vi "CC Focus GUI.vi"(9 "Standalone":bool=TRUE, 10 "Init Data":variant, 11 "Name":string) -> ()   [LabVIEW 2024]
uses:
  typedefs/CC enum Operation Mode.ctl
  Focus cluster Settings.ctl
  Focus Hardware Types.ctl
  Focus cluster Motion Settings.ctl
  Focus Class/Focus Class.lvclass
  Subsystems/SS typedef cluster Instrument Command Queue Data.ctl
  Subsystems/SS cluster Data Queue type.ctl
  Focus cluster MoveFocus Command Parameters.ctl
  FocusSimulator/FocusSimulator.lvclass
  C:/Development/Prime-RIMAS/Focus/Focus Class/Focus Class.lvclass
  NewFocus/NewFocus.lvclass
  Focus Class/Focus Class.lvclass/Focus Class.ctl
  hk-channel-class/hk-channel-class/HK Item/HK Channel cluster Telemetry Data.ctl
  hk-channel-class/hk-channel-class/HK Item/HK Channel enum Data Type.ctl
  hk-channel-class/hk-channel-class/HK Item/HK Item.lvclass
panel:
  out "Messages":string
  in  "Mode":T1
  in  "Tab Control":T2(tab)
  in  "Absolute":bool
  in  "Relative":bool
  in  "Steps":i32
  out "Controller Name":string
  in  "Select Motor (0:n-1)":i32 min=0 max=3 step=1
  out "Positions":i32[](array[slide]) scale=-10000.0..10000.0
  in  "Error":bool
  out "Homed":bool[](array[boolean])
  in  "STOP":bool
  out "Connected":bool
  in  "Close":bool
  in  "Home":bool
  in  "Reset Startup Positions":bool
  in  "Connect":bool
  in  "Focus Settings":T3
  in  "Power Up Positions":i32[](array[numeric])
  # "The focus motors adjust the position of the detectors. These motors should only be used at room temperatures. Adjustments to focus position is for maintenance personel only. There is nothing observers need to access."
  # "Click for info"
  # "We need to remember where we were last in case\npower cycled on NewFocus controller. Change\ncode to use saved positions only if controller reports\nall 0s for position."
  # "Factory Settings: \nVelocity 1750 Steps/sec\nAcceleration 100000 Steps/sec/sec"
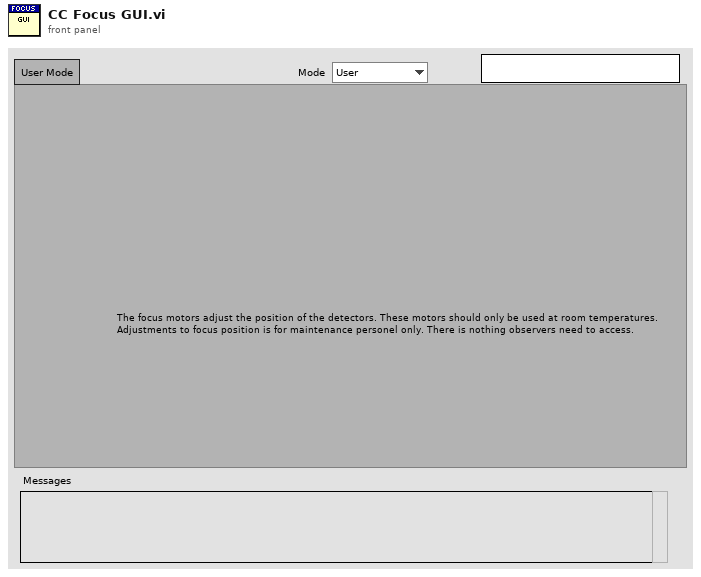
[diagram p1: front panel]
types:
  T1 = typedef "CC enum Operation Mode.ctl" = enum16{"User", "Engineering"}
  T2 = enum32{"User Mode", "Focus Motor", "Engineering"}
  T3 = typedef "Focus cluster Settings.ctl" = cluster{"Type":T4, "Motion Settings":T5, "Last Positions":i32[]}
  T4 = typedef "Focus Hardware Types.ctl" = enum16{"Simulated", "NewFocus"}
  T5 = typedef "Focus cluster Motion Settings.ctl" = cluster{"Steps Per Sec":i32, "Steps Per Sec 2":i32}
  T6 = typedef "SS typedef cluster Instrument Command Queue Data.ctl" = cluster{"Cmd":string, "Parameters":variant}
  T7 = typedef "Focus cluster MoveFocus Command Parameters.ctl" = cluster{"Motor":i32, "Position":i32}
  T8 = cluster{"state":refnum<user-event>, "Focus Settings":T3, "Focus Ref":refnum<class "Focus Class.lvclass">, "Error":errorcluster, "Msg":string, "Start Pos":i32[], "cmd q":refnum<queue>, "data q":refnum<queue>, "next poll":timestamp, "Cmd":T6, "move":T7, "Name":string}
  T9 = typedef "SS cluster Data Queue type.ctl" = cluster{"Source":string, "Type":string, "Data":variant}
  T10 = typedef "HK Item.lvclass/HK Channel enum Data Type.ctl" = enum16{"Floating Point", "Integer", "Enum", "String", "Waveform", "File"}
  T11 = typedef "HK Item.lvclass/HK Channel cluster Telemetry Data.ctl" = cluster{"Ch Names":string[], "Ch Values":dbl[], "Timestamp":timestamp, "Data Type":T10}
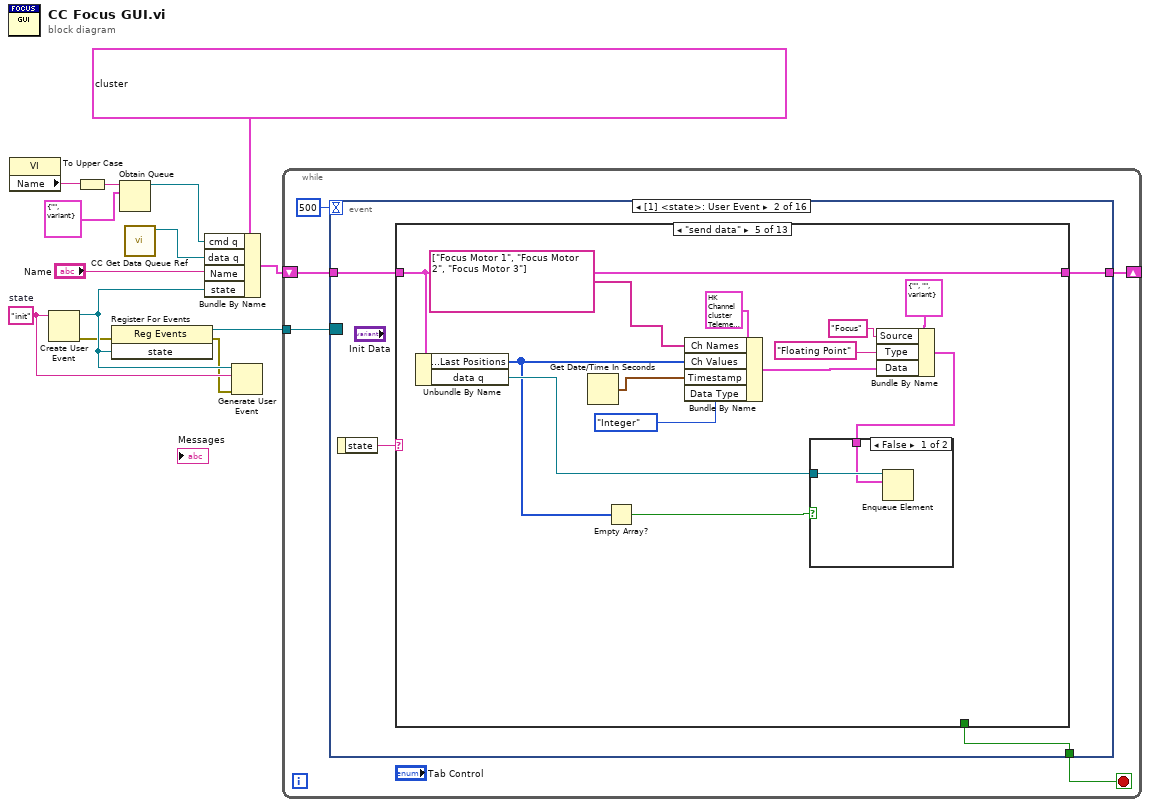
[diagram p0: block diagram]
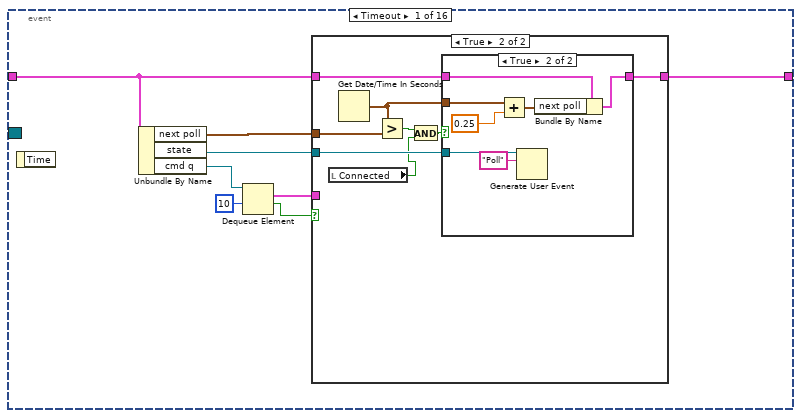
[diagram p2: hidden frame]
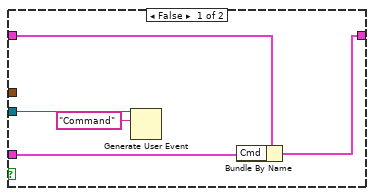
[diagram p3: hidden frame]
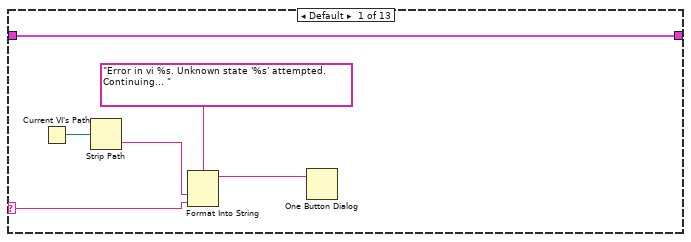
[diagram p5: hidden frame]
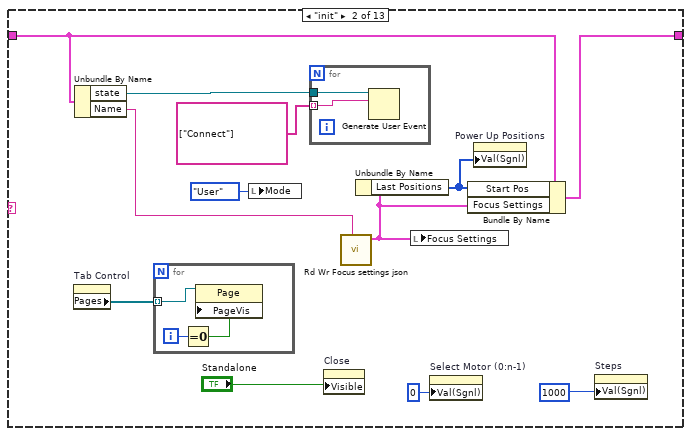
[diagram p6: hidden frame]
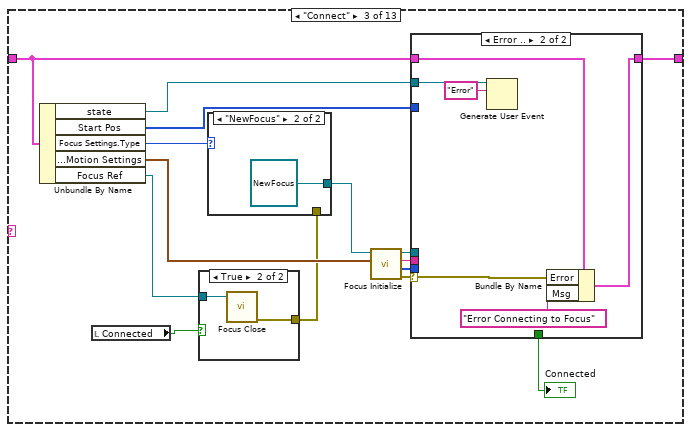
[diagram p7: hidden frame]
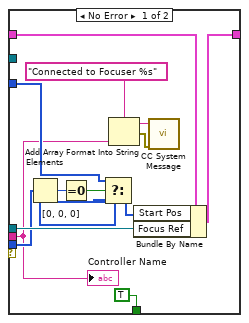
[diagram p9: hidden frame]
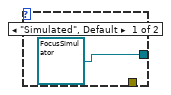
[diagram p10: hidden frame]
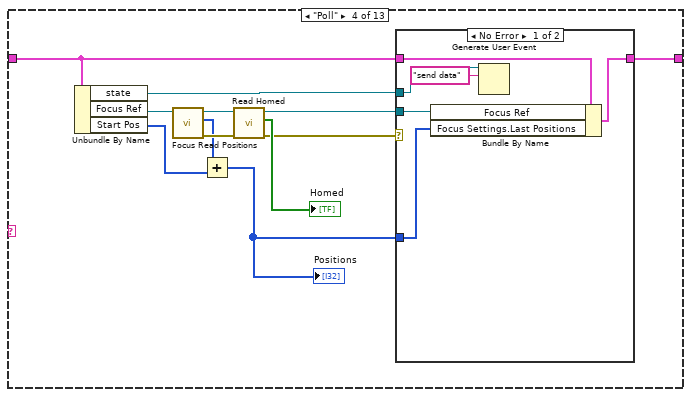
[diagram p11: hidden frame]
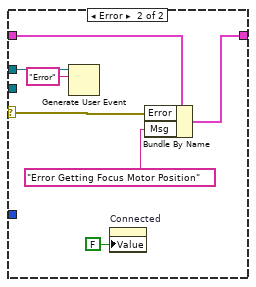
[diagram p12: hidden frame]
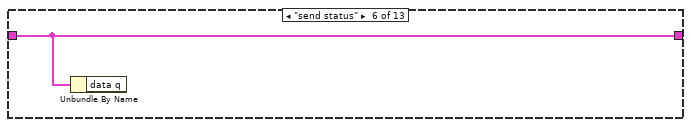
[diagram p14: hidden frame]
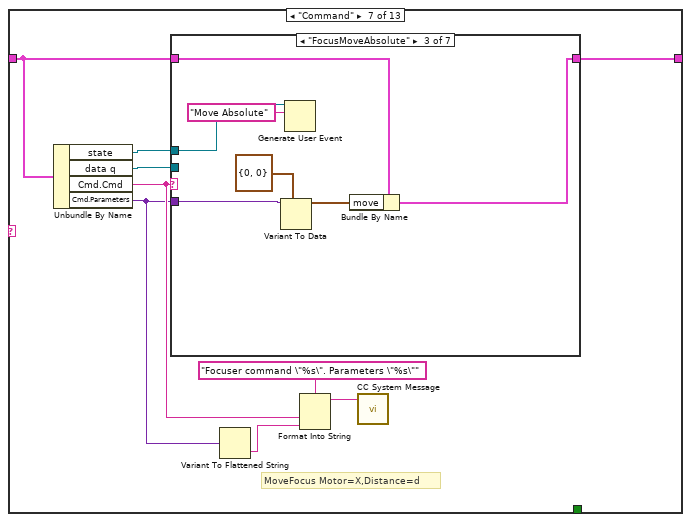
[diagram p15: hidden frame]
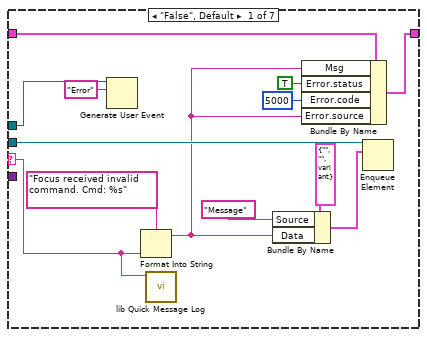
[diagram p16: hidden frame]
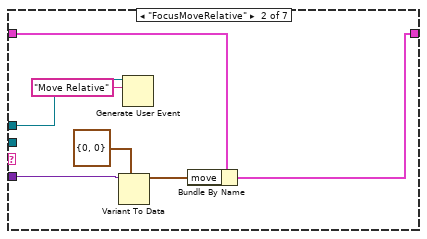
[diagram p17: hidden frame]
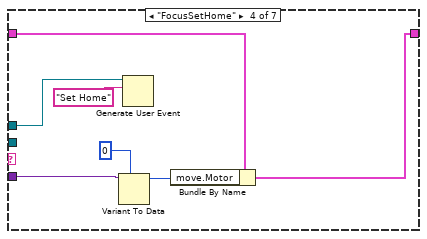
[diagram p18: hidden frame]
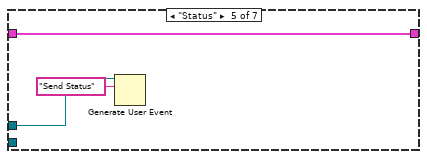
[diagram p19: hidden frame]
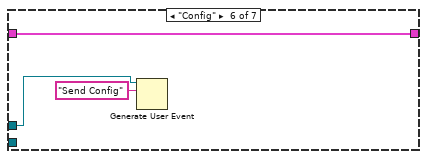
[diagram p20: hidden frame]
diagram:
  w9 = "init"  # state
  n1 = property class="VI"() -> ("Name"=w6:string)  [unwired: 2 in, 2 out]
  n2 = Create User Event(user event datatype=w9) -> (user event=w11:refnum<user-event>, error out=w7:errorcluster)  [unwired: 1 in]
  n3 = To Upper Case(1:w6) -> (0:w5:string)
  n4 = register-events(error in=w7, w11) -> (reference out=w10:refnum<event-registration>, error out=w8:errorcluster)  [unwired: 1 in]
  n5 = Obtain Queue(name (unnamed)=w5, element data type=T6 {"Cmd"="", "Parameters"=variant}) -> (queue out=w3:refnum<queue>)  [unwired: 3 in, 2 out]
  n6 = call "CC Get Data Queue Ref.vi"() -> ("Data Q"=w2:refnum<queue>)  [unwired: 10 in, 1 out]
  n7 = Bundle By Name(cluster=T8 {"state"=refnum, "Focus Settings"={"Type"=enum."Simulated", "Motion Settings"={"Steps Per Sec"=0, "Steps Per Sec 2"=0}, "Last Positions"=[]}, "Focus Ref"=refnum, "Error"={"status"=FALSE, "code"=0, "source"=""}, "Msg"="", "Start Pos"=[], "cmd q"=refnum, "data q"=refnum, "next poll"=timestamp(0 s since 1904-01-01), "Cmd"={"Cmd"="", "Parameters"=variant}, "move"={"Motor"=0, "Position"=0}, "Name"="NewFocus"}, "cmd q"=w3, "data q"=w2, "Name"="Name", "state"=w11) -> (w12:T8)
  n8 = Generate User Event(user event=w11, event data cluster=w9, error in=w8) -> ()  [unwired: 1 in, 2 out]
  n9 = while {
    tunnel: w10 -> [w18]
    shift-right: [w16] -> _
    shift-left: w12 -> [w17]
    stop <- w15 stop-if-true
    n10 = event shown="[1] <state>: User Event" {
      selector: w18 -> [_ _ _ _ _ _ _ _ _ _ _ _ _ _ _ _]
      dyn-events: _ -> [_ _ _ _ _ _ _ _ _ _ _ _ _ _ _ _]
      timeout: 500 -> [_ _ _ _ _ _ _ _ _ _ _ _ _ _ _ _]
      tunnel: w17 -> [w20 w50 w291 w303 w307 w310 w316 w319 w322 w325 w326 w336 w346 w349 w363 w366]
      tunnel: [w19 w49 w291 w304 w308 w311 w316 w319 w322 w325 w327 w337 w346 w350 w363 w366] -> w16
      tunnel: [_ w48 _ _ _ _ _ _ _ _ _ _ _ _ _ _] -> w15
      event Timeout {
        n11 = event-data() -> ()  [unwired: 1 in, 1 out]
        n12 = Unbundle By Name(w20) -> ("next poll"=w21:timestamp, "state"=w22:refnum<user-event>, "cmd q"=w26:refnum<queue>)
        n13 = Dequeue Element(queue=w26, timeout in ms (-1)=10) -> (element=w23:T6, timed out?=w24:bool)  [unwired: 1 in, 2 out]
        n14 = case shown="True" w24 {
          tunnel: w23 -> [w28 _]
          tunnel: w22 -> [w31 w36]
          tunnel: w20 -> [w29 w37]
          tunnel: [w27 w34] -> w19
          tunnel: w21 -> [_ w39]
          frame False {
            n15 = Generate User Event(user event=w31, event data cluster="Command" ("event data")) -> ()  [unwired: 2 in, 2 out]
            n16 = Bundle By Name(cluster=w29, "Cmd"=w28) -> (w27:T8)
          }
          frame True {
            n17 = local read "Connected"() -> (w32:bool)
            n18 = Get Date/Time In Seconds() -> (seconds since 1Jan1904=w35:timestamp)
            n19 = Greater?(x=w35, y=w39) -> (0:w38:bool)
            n20 = And(x=w38, y=w32) -> (x .and. y?=w33:bool)
            n21 = case shown="True" w33 {
              tunnel: w37 -> [w40 w47]
              tunnel: w36 -> [_ w46]
              tunnel: w35 -> [_ w45]
              tunnel: [w40 w42] -> w34
              frame False {
              }
              frame True {
                n22 = Add(x=w45, y=0.25) -> (x+y=w43:timestamp)
                n23 = Generate User Event(user event=w46, event data cluster="Poll" ("event data")) -> ()  [unwired: 2 in, 2 out]
                n24 = Bundle By Name(cluster=w47, "next poll"=w43) -> (w42:T8)
              }
            }
          }
        }
      }
      event User Event {
        n25 = event-data() -> ("state"=w51:string)  [unwired: 1 in]
        n26 = case shown="\"send data\"" w51 {
          selector: w51 -> [w56 _ _ _ _ _ _ _ _ _ _ _ _]
          tunnel: w50 -> [w52 w66 w85 w119 w151 w154 w160 w207 w218 w239 w260 w281 w288]
          tunnel: [w52 w67 w86 w118 w151 w154 w161 w208 w219 w240 w261 w281 w288] -> w49
          tunnel: [_ _ _ _ _ _ _ _ _ _ _ TRUE _] -> w48
          frame Default {
            n27 = Current VI's Path() -> (path=w55:path)
            n28 = Strip Path(path=w55) -> (name=w54:string)  [unwired: 1 out]
            n29 = Format Into String(format string="Error in vi %s. Unknown state '%s' attempted. Continuing... ", w54, w56) -> (resulting string=w53:string)  [unwired: 2 in, 1 out]
            n30 = One Button Dialog(message=w53) -> ()  [unwired: 1 in, 1 out]
          }
          frame "init" {
            n31 = property on="Tab Control" class="TabCtl (strict)"() -> ("Pages"=w58:refnum<vi>[])  [unwired: 2 in, 2 out]
            n32 = Unbundle By Name(w66) -> ("state"=w69:refnum<user-event>, "Name"=w60:string)
            n33 = for {
              tunnel: w58 -> [w72] mode=indexing
              i -> [w71]
              n34 = Equal To 0?(x=w71) -> (x = 0?=w70:bool)
              n35 = property class="Page"(reference=w72, "PageVis"=w70) -> ()  [unwired: 1 in, 2 out]
            }
            n36 = local write "Mode"(CC_enum_Operation_Mode."User" ("Mode")) -> ()
            n37 = for {
              tunnel: w69 -> [w74]
              tunnel: string[] ["Connect"] -> [w73] mode=indexing
              n38 = Generate User Event(user event=w74, event data cluster=w73) -> ()  [unwired: 2 in, 2 out]
            }
            n39 = property on="Close" class="Bool"("Visible"="Standalone") -> ()  [unwired: 2 in, 2 out]
            n40 = call "Rd Wr Focus settings json.vi"("Focus Name"=w60) -> ("Focus Settings"=w62:T3)  [unwired: 9 in, 1 out]
            n41 = Unbundle By Name(w62) -> ("Last Positions"=w61:i32[])
            n42 = local write "Focus Settings"(w62) -> ()
            n43 = property on="Select Motor (0:n-1)" class="DigNum (strict)"("Val(Sgnl)"=0 ("Value (Signaling)")) -> ()  [unwired: 2 in, 2 out]
            n44 = Bundle By Name(cluster=w66, "Start Pos"=w61, "Focus Settings"=w62) -> (w67:T8)
            n45 = property on="Power Up Positions" class="Arr (strict)"("Val(Sgnl)"=w61) -> ()  [unwired: 2 in, 2 out]
            n46 = property on="Steps" class="DigNum (strict)"("Val(Sgnl)"=1000 ("Steps")) -> ()  [unwired: 2 in, 2 out]
          }
          frame "Connect" {
            n47 = Unbundle By Name(w85) -> ("state"=w82:refnum<user-event>, "Start Pos"=w75:i32[], "Focus Settings.Type"=w89:T4, "Focus Settings.Motion Settings"=w84:T5, "Focus Ref"=w78:refnum<class "Focus Class.lvclass">)
            n48 = local read "Connected"() -> (w79:bool)
            n49 = case shown="True" w79 {
              tunnel: w78 -> [_ w91]
              tunnel: [_ w90] -> w77
              frame False {
              }
              frame True {
                n50 = call-dynamic "Focus Close.vi"("Focus Class in"=w91) -> ("error out"=w90:errorcluster)  [unwired: 9 in, 1 out]
              }
            }
            n51 = case shown="\"NewFocus\"" w89 {
              tunnel: [refnum<class "FocusSimulator.lvclass"> refnum ("FocusSimulator.lvclass") refnum<class "NewFocus.lvclass"> refnum ("NewFocus.lvclass")] -> w88
              tunnel: w77 -> [_ _]
              frame "Simulated", Default {
              }
              frame "NewFocus" {
              }
            }
            n52 = call-dynamic "Focus Initialize.vi"("Motion Settings"=w84, "Focus Class in"=w88) -> ("error out"=w83:errorcluster, "Motor Positions"=w76:i32[], "Device Name"=w81:string, "Focus Class out"=w87:refnum<class "Focus Class.lvclass">)  [unwired: 6 in]
            n53 = case shown="Error .." w83 {
              selector: w83 -> [_ w110]
              tunnel: w87 -> [w105 _]
              tunnel: [w104 w109] -> w86
              tunnel: w85 -> [w103 w111]
              tunnel: w82 -> [_ w108]
              tunnel: w81 -> [w92 _]
              tunnel: [TRUE _] -> w80
              tunnel: w76 -> [w101 _]
              tunnel: w75 -> [w97 _]
              frame No Error {
                n54 = Add Array Elements(numeric array=w101) -> (sum=w100:i32)
                n55 = Equal To 0?(x=w100) -> (x = 0?=w99:bool)
                n56 = Select(t=w97, s=w99, f=i32[] [0, 0, 0] ("t")) -> (s? t:f=w98:i32[])
                n57 = Format Into String(format string="Connected to Focuser %s", w92) -> (resulting string=w93:string, error out=w95:errorcluster)  [unwired: 2 in]
                n58 = Bundle By Name(cluster=w103, "Start Pos"=w98, "Focus Ref"=w105) -> (w104:T8)
                n59 = call "CC System Message.vi"("error in (no error)"=w95, "Message"=w93) -> ()  [unwired: 9 in, 1 out]
                "Controller Name" <- w92
              }
              frame Error {
                n60 = Generate User Event(user event=w108, event data cluster="Error" ("event data")) -> ()  [unwired: 2 in, 2 out]
                n61 = Bundle By Name(cluster=w111, "Error"=w110, "Msg"="Error Connecting to Focus") -> (w109:T8)
              }
            }
            "Connected" <- w80
          }
          frame "Poll" {
            n62 = Unbundle By Name(w119) -> ("state"=w120:refnum<user-event>, "Focus Ref"=w125:refnum<class "Focus Class.lvclass">, "Start Pos"=w114:i32[])
            n63 = call-dynamic "Focus Read Positions.vi"("Focus Class in"=w125) -> ("error out"=w123:errorcluster, "Motor Positions"=w116:i32[], "Focus Class out"=w124:refnum<class "Focus Class.lvclass">)  [unwired: 8 in]
            n64 = Add(x=w116, y=w114) -> (x+y=w115:i32[])
            "Positions" <- w115
            n65 = call "Read Homed.vi"("error in (no error)"=w123, "Focus Class in"=w124) -> ("error out"=w121:errorcluster, "Homed"=→"Homed":bool[], "Focus Class out"=w117:refnum<class "Focus Class.lvclass">)  [unwired: 7 in]
            n66 = case shown="No Error" w121 {
              selector: w121 -> [_ w135]
              tunnel: w120 -> [w127 w137]
              tunnel: w119 -> [w129 w138]
              tunnel: [w130 w133] -> w118
              tunnel: w117 -> [w131 _]
              tunnel: w115 -> [w128 _]
              frame No Error {
                n67 = Bundle By Name(cluster=w129, "Focus Ref"=w131, "Focus Settings.Last Positions"=w128) -> (w130:T8)
                n68 = Generate User Event(user event=w127, event data cluster="send data" ("event data")) -> ()  [unwired: 2 in, 2 out]
              }
              frame Error {
                n69 = Generate User Event(user event=w137, event data cluster="Error" ("event data")) -> ()  [unwired: 2 in, 2 out]
                n70 = property on="Connected" class="Bool (strict)"("Value"=FALSE ("Connected")) -> ()  [unwired: 2 in, 2 out]
                n71 = Bundle By Name(cluster=w138, "Error"=w135, "Msg"="Error Getting Focus Motor Position") -> (w133:T8)
              }
            }
          }
          frame "send data" {
            n72 = Unbundle By Name(w151) -> ("Focus Settings.Last Positions"=w140:i32[], "data q"=w146:refnum<queue>)
            n73 = Get Date/Time In Seconds() -> (seconds since 1Jan1904=w148:timestamp)
            n74 = Empty Array?(array=w140) -> (empty?=w139:bool)
            n75 = Bundle By Name(cluster=T11 {"Ch Names"=[], "Ch Values"=[], "Timestamp"=timestamp(0 s since 1904-01-01), "Data Type"=enum."Floating Point"}, "Ch Names"=string[] ["Focus Motor 1", "Focus Motor 2", "Focus Motor 3"], "Ch Values"=w140, "Timestamp"=w148, "Data Type"=HK_Channel_enum_Data_Type."Integer") -> (w142:T11)
            n76 = Bundle By Name(cluster=T9 {"Source"="", "Type"="", "Data"=variant} ("element"), "Source"="Focus", "Type"="Floating Point" ("Data Type"), "Data"=w142) -> (w141:T9)
            n77 = case shown="False" w139 {
              tunnel: w146 -> [w153 _]
              tunnel: w141 -> [w152 _]
              frame False {
                n78 = Enqueue Element(queue=w153, element=w152) -> ()  [unwired: 2 in, 3 out]
              }
              frame True {
              }
            }
          }
          frame "send status" {
            n79 = Unbundle By Name(w154) -> ()  [unwired: 1 out]
          }
          frame "Command" {
            # "MoveFocus Motor=X,Distance=d"
            n80 = Unbundle By Name(w160) -> ("state"=w162:refnum<user-event>, "data q"=w163:refnum<queue>, "Cmd.Cmd"=w157:string, "Cmd.Parameters"=w156:variant)
            n81 = case shown="\"FocusMoveAbsolute\"" w157 {
              selector: w157 -> [w171 _ _ _ _ _ _]
              tunnel: w163 -> [w176 _ _ _ _ _ _]
              tunnel: w156 -> [_ w183 w190 w197 _ _ _]
              tunnel: w162 -> [w167 w179 w186 w194 w200 w202 w206]
              tunnel: w160 -> [w170 w181 w188 w196 w198 w201 w204]
              tunnel: [w165 w180 w187 w195 w198 w201 w204] -> w161
              frame "False", Default {
                n82 = Generate User Event(user event=w167, event data cluster="Error" ("event data")) -> ()  [unwired: 2 in, 2 out]
                n83 = Format Into String(format string="Focus received invalid command. Cmd: %s", w171) -> (resulting string=w164:string)  [unwired: 2 in, 1 out]
                n84 = call "lib Quick Message Log.vi"("Message"=w171) -> ()  [unwired: 9 in, 2 out]
                n85 = Bundle By Name(cluster=T9 {"Source"="", "Type"="", "Data"=variant} ("element"), "Source"="Message" ("Data Type"), "Data"=w164) -> (w172:T9)
                n86 = Bundle By Name(cluster=w170, "Msg"=w164, "Error.status"=TRUE ("error.status"), "Error.code"=5000 ("error.code"), "Error.source"=w164) -> (w165:T8)
                n87 = Enqueue Element(queue=w176, element=w172) -> ()  [unwired: 2 in, 3 out]
              }
              frame "FocusMoveRelative" {
                n88 = Variant To Data(type=T7 {"Motor"=0, "Position"=0}, Variant=w183) -> (data=w177:T7)  [unwired: 1 in, 1 out]
                n89 = Generate User Event(user event=w179, event data cluster="Move Relative" ("event data")) -> ()  [unwired: 2 in, 2 out]
                n90 = Bundle By Name(cluster=w181, "move"=w177) -> (w180:T8)
              }
              frame "FocusMoveAbsolute" {
                n91 = Variant To Data(type=T7 {"Motor"=0, "Position"=0}, Variant=w190) -> (data=w184:T7)  [unwired: 1 in, 1 out]
                n92 = Generate User Event(user event=w186, event data cluster="Move Absolute" ("event data")) -> ()  [unwired: 2 in, 2 out]
                n93 = Bundle By Name(cluster=w188, "move"=w184) -> (w187:T8)
              }
              frame "FocusSetHome" {
                n94 = Variant To Data(type=0 ("move.Motor"), Variant=w197) -> (data=w192:i32)  [unwired: 1 in, 1 out]
                n95 = Generate User Event(user event=w194, event data cluster="Set Home" ("event data")) -> ()  [unwired: 2 in, 2 out]
                n96 = Bundle By Name(cluster=w196, "move.Motor"=w192) -> (w195:T8)
              }
              frame "Status" {
                n97 = Generate User Event(user event=w200, event data cluster="Send Status" ("event data")) -> ()  [unwired: 2 in, 2 out]
              }
              frame "Config" {
                n98 = Generate User Event(user event=w202, event data cluster="Send Config" ("event data")) -> ()  [unwired: 2 in, 2 out]
              }
              frame "Shutdown" {
                n99 = Generate User Event(user event=w206, event data cluster="Shutdown" ("event data")) -> ()  [unwired: 2 in, 2 out]
              }
            }
            n100 = Variant To Flattened String(Variant=w156) -> (data string=w155:string)  [unwired: 1 out]
            n101 = Format Into String(format string="Focuser command \"%s\". Parameters \"%s\"", w157, w155) -> (resulting string=w158:string)  [unwired: 2 in, 1 out]
            n102 = call "CC System Message.vi"("Message"=w158) -> ()  [unwired: 10 in, 1 out]
          }
          frame "Stop" {
            n103 = Unbundle By Name(w207) -> ("Focus Ref"=w213:refnum<class "Focus Class.lvclass">, "move.Motor"=w211:i32)
            n104 = call-dynamic "Focus Stop.vi"("Motor (0:n-1)"=w211, "Focus Class in"=w213) -> ("Focus Class out"=w209:refnum<class "Focus Class.lvclass">)  [unwired: 8 in, 1 out]
            n105 = Bundle By Name(cluster=w207, "Focus Ref"=w209) -> (w208:T8)
            n106 = Format Into String(format string="Focuser stop motor %d" ("Message"), w211) -> (resulting string=w210:string)  [unwired: 2 in, 1 out]
            n107 = call "CC System Message.vi"("Message"=w210) -> ()  [unwired: 10 in, 1 out]
          }
          frame "Set Home" {
            n108 = Unbundle By Name(w218) -> ("state"=w220:refnum<user-event>, "Focus Ref"=w222:refnum<class "Focus Class.lvclass">, "move.Motor"=w214:i32)
            n109 = call-dynamic "Focus Set Home.vi"("Motor (0:n-1)"=w214, "Focus Class in"=w222) -> ("error out"=w221:errorcluster, "Focus Class out"=w217:refnum<class "Focus Class.lvclass">)  [unwired: 8 in]
            n110 = case shown="No Error" w221 {
              selector: w221 -> [_ w230]
              tunnel: w220 -> [_ w233]
              tunnel: w218 -> [w225 w231]
              tunnel: [w224 w229] -> w219
              tunnel: w214 -> [_ w227]
              tunnel: w217 -> [w223 _]
              frame No Error {
                n111 = Bundle By Name(cluster=w225, "Focus Ref"=w223) -> (w224:T8)
              }
              frame Error {
                n112 = Generate User Event(user event=w233, event data cluster="Error" ("event data")) -> ()  [unwired: 2 in, 2 out]
                n113 = Format Into String(format string="Error Setting Home Position on Focus Motor %d" ("Msg"), w227) -> (resulting string=w226:string)  [unwired: 2 in, 1 out]
                n114 = Bundle By Name(cluster=w231, "Error"=w230, "Msg"=w226) -> (w229:T8)
              }
            }
            n115 = Format Into String(format string="Focuser home motor %d" ("Message"), w214) -> (resulting string=w215:string)  [unwired: 2 in, 1 out]
            n116 = call "CC System Message.vi"("Message"=w215) -> ()  [unwired: 10 in, 1 out]
          }
          frame "Move Relative" {
            n117 = Unbundle By Name(w239) -> ("state"=w241:refnum<user-event>, "Focus Ref"=w243:refnum<class "Focus Class.lvclass">, "move.Motor"=w235:i32, "move.Position"=w234:i32)
            n118 = call-dynamic "Focus Move Relative.vi"("Counts"=w234, "Motor (0:n-1)"=w235, "Focus Class in"=w243) -> ("error out"=w242:errorcluster, "Focus Class out"=w238:refnum<class "Focus Class.lvclass">)  [unwired: 7 in]
            n119 = case shown="No Error" w242 {
              selector: w242 -> [_ w251]
              tunnel: w241 -> [_ w254]
              tunnel: w239 -> [w246 w252]
              tunnel: [w245 w250] -> w240
              tunnel: w235 -> [_ w248]
              tunnel: w238 -> [w244 _]
              frame No Error {
                n120 = Bundle By Name(cluster=w246, "Focus Ref"=w244) -> (w245:T8)
              }
              frame Error {
                n121 = Generate User Event(user event=w254, event data cluster="Error" ("event data")) -> ()  [unwired: 2 in, 2 out]
                n122 = Format Into String(format string="Error Moving motor %d" ("Msg"), w248) -> (resulting string=w247:string)  [unwired: 2 in, 1 out]
                n123 = Bundle By Name(cluster=w252, "Error"=w251, "Msg"=w247) -> (w250:T8)
              }
            }
            n124 = Format Into String(format string="Focuser relative move motor %d to position %d" ("Message"), w235, w234) -> (resulting string=w236:string)  [unwired: 2 in, 1 out]
            n125 = call "CC System Message.vi"("Message"=w236) -> ()  [unwired: 10 in, 1 out]
          }
          frame "Move Absolute" {
            n126 = Unbundle By Name(w260) -> ("state"=w262:refnum<user-event>, "Focus Ref"=w264:refnum<class "Focus Class.lvclass">, "move.Motor"=w256:i32, "move.Position"=w255:i32)
            n127 = call-dynamic "Focus Move Absolute.vi"("Position"=w255, "Motor (0:n-1)"=w256, "Focus Class in"=w264) -> ("error out"=w263:errorcluster, "Focus Class out"=w259:refnum<class "Focus Class.lvclass">)  [unwired: 7 in]
            n128 = case shown="No Error" w263 {
              selector: w263 -> [_ w272]
              tunnel: w262 -> [_ w275]
              tunnel: w260 -> [w267 w273]
              tunnel: [w265 w271] -> w261
              tunnel: w256 -> [_ w269]
              tunnel: w259 -> [w266 _]
              frame No Error {
                n129 = Bundle By Name(cluster=w267, "Focus Ref"=w266) -> (w265:T8)
              }
              frame Error {
                n130 = Generate User Event(user event=w275, event data cluster="Error" ("event data")) -> ()  [unwired: 2 in, 2 out]
                n131 = Format Into String(format string="Error Moving motor %d" ("Msg"), w269) -> (resulting string=w268:string)  [unwired: 2 in, 1 out]
                n132 = Bundle By Name(cluster=w273, "Error"=w272, "Msg"=w268) -> (w271:T8)
              }
            }
            n133 = Format Into String(format string="Focuser absoluite move motor %d to position %d" ("Message"), w256, w255) -> (resulting string=w257:string)  [unwired: 2 in, 1 out]
            n134 = call "CC System Message.vi"("Message"=w257) -> ()  [unwired: 10 in, 1 out]
          }
          frame "Shutdown" {
            n135 = Unbundle By Name(w281) -> ("Focus Settings"=w278:T3, "Focus Ref"=w280:refnum<class "Focus Class.lvclass">)
            n136 = call-dynamic "Focus Close.vi"("Focus Class in"=w280) -> ()  [unwired: 9 in, 2 out]
            n137 = call "Rd Wr Focus settings json.vi"("Write? (F:Read)"=TRUE, "Focus Settings"=w278) -> ()  [unwired: 8 in, 2 out]
            n138 = call "CC System Message.vi"("Message"="Focuser shutdown.") -> ()  [unwired: 10 in, 1 out]
          }
          frame "Error" {
            n139 = Unbundle By Name(w288) -> ("Error.status"=w287:bool, "Error.source"=w282:string, "Name"=w283:string)
            n140 = local write "Error"(w287) -> ()
            n141 = Format Into String(format string="Error connecting to focus motors %s. Error message: %s", w283, w282) -> (resulting string=w284:string, error out=w286:errorcluster)  [unwired: 2 in]
            n142 = call "CC System Message.vi"("error in (no error)"=w286, "Message"=w284) -> ()  [unwired: 9 in, 1 out]
          }
        }
      }
      event Value Change {
        n143 = event-data() -> ()  [unwired: 1 in, 6 out]
        n144 = property on="Tab Control" class="TabCtl (strict)"() -> ("Pages"=w289:refnum<vi>[])  [unwired: 2 in, 2 out]
        n145 = case shown="\"Engineering\"" "Mode" {
          tunnel: w289 -> [w292 w296]
          frame "User", Default {
            n146 = for {
              tunnel: w292 -> [w295] mode=indexing
              i -> [w294]
              n147 = Equal To 0?(x=w294) -> (x = 0?=w293:bool)
              n148 = property class="Page"(reference=w295, "PageVis"=w293) -> ()  [unwired: 1 in, 2 out]
            }
          }
          frame "Engineering" {
            n149 = for {
              tunnel: w296 -> [w298] mode=indexing
              n150 = property class="Page"(reference=w298, "PageVis"=TRUE ("Page Visible")) -> ()  [unwired: 1 in, 2 out]
            }
          }
        }
      }
      event Value Change {
        n151 = event-data() -> ()  [unwired: 1 in, 6 out]
        n152 = Unbundle By Name(w303) -> ("state"=w302:refnum<user-event>)
        n153 = for {
          tunnel: w302 -> [w306]
          tunnel: string[] ["Connect"] -> [w305] mode=indexing
          n154 = Generate User Event(user event=w306, event data cluster=w305) -> ()  [unwired: 2 in, 2 out]
        }
        n155 = call "Rd Wr Focus settings json.vi"("Write? (F:Read)"=TRUE, "Focus Settings"="Focus Settings") -> ()  [unwired: 8 in, 2 out]
        n156 = Bundle By Name(cluster=w303, "Focus Settings"="Focus Settings") -> (w304:T8)
      }
      event "Select Motor (0:n-1)": Value Change {
        n157 = event-data() -> ()  [unwired: 1 in, 6 out]
        n158 = Bundle By Name(cluster=w307, "move.Motor"="Select Motor (0:n-1)") -> (w308:T8)
      }
      event "Steps": Value Change {
        n159 = event-data() -> ("NewVal"=w312:i32)  [unwired: 1 in]
        n160 = Bundle By Name(cluster=w310, "move.Position"=w312) -> (w311:T8)
      }
      event "Connect": Value Change {
        n161 = event-data() -> ()  [unwired: 1 in, 6 out]
        n162 = Unbundle By Name(w316) -> ("state"=w314:refnum<user-event>, "Focus Ref"=w315:refnum<class "Focus Class.lvclass">)
        n163 = call-dynamic "Focus Close.vi"("Focus Class in"=w315) -> ()  [unwired: 9 in, 2 out]
        n164 = Generate User Event(user event=w314, event data cluster="Connect" ("event data")) -> ()  [unwired: 2 in, 2 out]
      }
      event "Home": Value Change {
        n165 = event-data() -> ()  [unwired: 1 in, 6 out]
        n166 = Unbundle By Name(w319) -> ("state"=w318:refnum<user-event>)
        n167 = Generate User Event(user event=w318, event data cluster="Set Home" ("event data")) -> ()  [unwired: 2 in, 2 out]
      }
      event "Relative": Value Change {
        n168 = event-data() -> ()  [unwired: 1 in, 6 out]
        n169 = Unbundle By Name(w322) -> ("state"=w321:refnum<user-event>)
        n170 = Generate User Event(user event=w321, event data cluster="Move Relative" ("event data")) -> ()  [unwired: 2 in, 2 out]
      }
      event "Absolute": Value Change {
        n171 = event-data() -> ()  [unwired: 1 in, 6 out]
        n172 = Unbundle By Name(w325) -> ("state"=w324:refnum<user-event>)
        n173 = Generate User Event(user event=w324, event data cluster="Move Absolute" ("event data")) -> ()  [unwired: 2 in, 2 out]
      }
      event "Power Up Positions": Value Change {
        n174 = event-data() -> ("NewVal"=w331:i32[])  [unwired: 1 in]
        n175 = Array Size(array=w331) -> (size(s)=w330:i32)
        n176 = Equal?(x=w330, y=3) -> (x = y?=w328:bool)
        n177 = case shown="False" w328 {
          tunnel: w326 -> [w334 w335]
          tunnel: [w332 w335] -> w327
          frame False {
            n178 = Bundle By Name(cluster=w334, "Start Pos"=i32[] [0, 0, 0] ("NewVal")) -> (w332:T8)
          }
          frame True {
          }
        }
      }
      event "Reset Startup Positions": Value Change {
        n179 = event-data() -> ()  [unwired: 1 in, 6 out]
        n180 = Array Size(array="Power Up Positions") -> (size(s)=w343:i32)
        n181 = Equal?(x=w343, y=3) -> (x = y?=w341:bool)
        n182 = Select(t="Power Up Positions", s=w341, f=i32[] [0, 0, 0] ("NewVal")) -> (s? t:f=w338:i32[])
        n183 = Bundle By Name(cluster=w336, "Start Pos"=w338) -> (w337:T8)
      }
      event "STOP": Value Change {
        n184 = event-data() -> ()  [unwired: 1 in, 6 out]
        n185 = Unbundle By Name(w346) -> ("state"=w345:refnum<user-event>)
        n186 = Generate User Event(user event=w345, event data cluster="Stop" ("event data")) -> ()  [unwired: 2 in, 2 out]
      }
      event "Error": Value Change {
        n187 = event-data() -> ("CtlRef"=w348:refnum<vi>)  [unwired: 1 in]
        n188 = Unbundle By Name(w349) -> ("Msg"=w351:string, "Error.code"=w356:i32, "Error.source"=w355:string, "Error.status"=w354:bool)
        n189 = Format Into String(format string="An error occurred during %s. \nError Number: %d\nError message: %s", w351, w356, w355) -> (resulting string=w353:string)  [unwired: 2 in, 1 out]
        n190 = call "Display Message to User"("Enable"=w354, "Message"=w353) -> ("error out"=w352:errorcluster, "Close"=w347:bool)  [unwired: 8 in]
        n191 = case shown="False" w347 {
          tunnel: w349 -> [w360 w361]
          tunnel: [w358 w361] -> w350
          tunnel: w352 -> [w359 _]
          frame False {
            n192 = Bundle By Name(cluster=w360, "Error"=w359) -> (w358:T8)
          }
          frame True {
          }
        }
        n193 = property class="Bool (strict)"(reference=w348, "Value"=w347) -> ()  [unwired: 1 in, 2 out]
      }
      event "Standalone": Value Change {
        n194 = event-data() -> ("NewVal"=w362:bool)  [unwired: 1 in]
        n195 = property on="Close" class="Bool"("Visible"=w362) -> ()  [unwired: 2 in, 2 out]
      }
      event "Close": Value Change {
        n196 = event-data() -> ()  [unwired: 1 in, 6 out]
        n197 = Unbundle By Name(w366) -> ("state"=w365:refnum<user-event>)
        n198 = Generate User Event(user event=w365, event data cluster="Shutdown" ("event data")) -> ()  [unwired: 2 in, 2 out]
      }
    }
  }
